vi "Actor Enqueuers FGV.vi"(5 "Enqueuer":T1=enum."CRDS", 7 "State":enum16{"Store", "Send MSG"}(ring)=enum."Send MSG", 8 "error in":errorcluster, 10 "MSG":refnum<class "Message.lvclass">, 11 "Enqueuer Map":variant) -> (0 "error out":errorcluster)   [LabVIEW 2014, in "Controller.lvlib" / "Controller.lvclass"]
doc: "This is a functional global variable for facillitating communication between web services and the te instruments that are under the control of the controller actor. This allows the web services to enqueue messages to be handled by the specific instruments directly rather than requiring further routing. This should cut down on the messages required by the system, allowing the web services to act as an extension of the controller application itself."
uses:
  Controller.lvclass
  <vilib>/ActorFramework/Message/Message.lvclass
  Controls/Enqueuer Enum.ctl
  <vilib>/ActorFramework/Message Enqueuer/Message Enqueuer.lvclass
  <vilib>/ActorFramework/Message Enqueuer/Message Enqueuer.lvclass/Message Enqueuer.ctl
  <vilib>/ActorFramework/Message Priority Queue/Priority Enqueue.vi
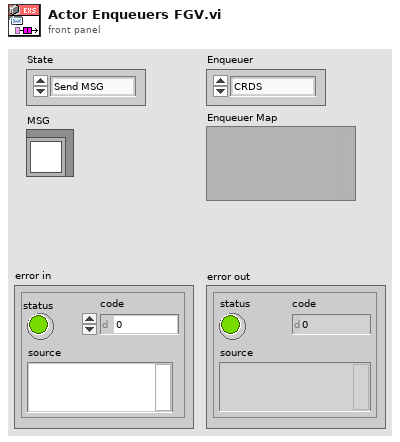
[diagram p1: front panel]
types:
  T1 = typedef "Controller.lvlib/Controller.lvclass/Enqueuer Enum.ctl" = enum8{"PAS", "CRDS", "File", "O3Lamp"}
  T2 = cluster{"Message Enqueuer out":refnum<class "Message Enqueuer.lvclass">, bool}
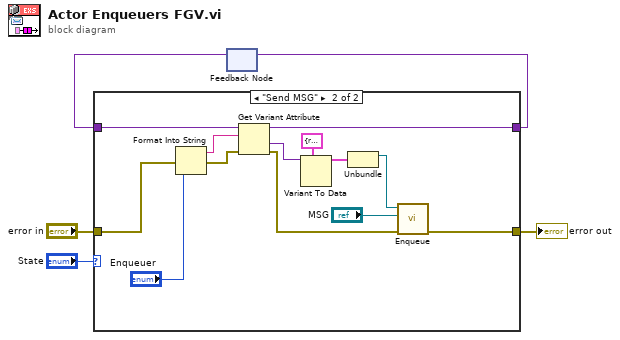
[diagram p0: block diagram]
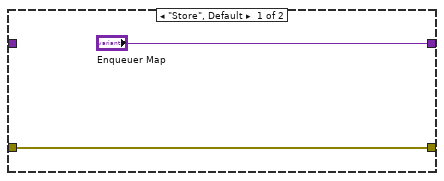
[diagram p2: hidden frame]
diagram:
  n1 = feedback #1() -> (w1:variant)  [unwired: 1 in]
  n2 = case shown="\"Send MSG\"" "State" {
    tunnel: [w7 w20] -> w4
    tunnel: "error in" -> [w7 w10]
    tunnel: w1 -> [_ w17]
    tunnel: ["Enqueuer Map" w13] -> w2
    frame "Store", Default {
    }
    frame "Send MSG" {
      n3 = Format Into String(error in=w10, "Enqueuer") -> (resulting string=w16:string, error out=w9:errorcluster)  [unwired: 2 in]
      n4 = Get Variant Attribute(Variant=w17, name=w16, error in=w9) -> (duplicate Variant=w13:variant, value=w15:variant, error out=w8:errorcluster)  [unwired: 1 in, 1 out]
      n5 = Variant To Data(type=T2 {"Message Enqueuer out"=refnum, TRUE}, Variant=w15) -> (data=w12:T2)  [unwired: 1 in, 1 out]
      n6 = Unbundle(w12) -> ("Message Enqueuer out"=w11:refnum<class "Message Enqueuer.lvclass">)  [unwired: 1 out]
      n7 = call <vilib>:"Enqueue.vi"("error in (no error)"=w8, "Message"="MSG", "Message Enqueuer in"=w11) -> ("error out"=w20:errorcluster)  [unwired: 7 in, 1 out]
    }
  }
  "error out" <- w4
  n8 = feedback-in #1(w2) -> ()
